vi "simulate_capslock_main.vi"(0 "Input_String":string) -> ()   [LabVIEW 2020]
doc: "This VI is used to display the alphabets capitalized if entered small and vice versa."
panel:
  # "Operation:\n\nIn this when the input string is small then the \noutput shows it capitalized and vice versa"
  # "IF you enter 'A'' it will display 'a'"
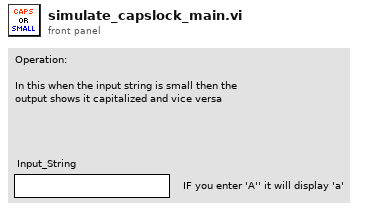
[diagram p1: front panel]
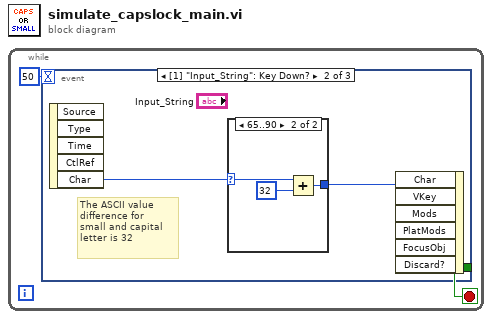
[diagram p0: block diagram]
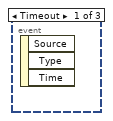
[diagram p2: hidden frame]
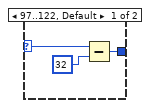
[diagram p3: hidden frame]
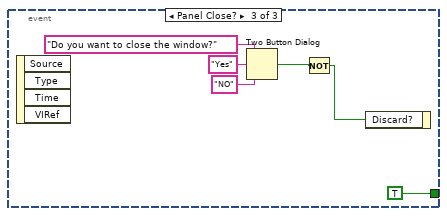
[diagram p4: hidden frame]
diagram:
  n1 = while {
    stop <- w1 stop-if-true
    n2 = event shown="[1] \"Input_String\": Key Down?" {
      selector: _ -> [_ _ _]
      dyn-events: _ -> [_ _ _]
      timeout: 50 -> [_ _ _]
      tunnel: [_ _ TRUE] -> w1
      event Timeout {
        n3 = event-data() -> ()  [unwired: 1 in, 3 out]
      }
      event "Input_String": Key Down? {
        # "The ASCII value \ndifference for \nsmall and capital \nletter is 32"
        n4 = event-data() -> ("Char"=w4:i16)  [unwired: 1 in, 4 out]
        n5 = case shown="65..90" w4 {
          selector: w4 -> [w7 w10]
          tunnel: [w5 w8] -> w3
          frame 97..122, Default {
            n6 = Subtract(x=w7, y=i16 32) -> (x-y=w5:i16)
          }
          frame 65..90 {
            n7 = Add(x=w10, y=i16 32) -> (x+y=w8:i16)
          }
        }
        n8 = event-data("Char"=w3) -> ()  [unwired: 6 in, 1 out]
      }
      event Panel Close? {
        n9 = event-data() -> ()  [unwired: 1 in, 4 out]
        n10 = Two Button Dialog(message="Do you want to close the window?", 1:"NO" ("F button name (\"Cancel\")"), 2:"Yes" ("T button name (\"OK\")")) -> (T button?=w12:bool)
        n11 = Not(x=w12) -> (.not. x?=w11:bool)
        n12 = event-data("Discard?"=w11) -> ()  [unwired: 1 in, 1 out]
      }
    }
  }
